vi "Read State.vi"(8 "error in (no error)":errorcluster, 11 "GoalKickKeeperTacticVSS in":refnum<class "GoalKickKeeperTacticVSS.lvclass">) -> (0 "error out":errorcluster, 2 "State":enum16{"GoToBallKeeper", "Kick", "Exit"}(ring), 3 "GoalKickKeeperTacticVSS out":refnum<class "GoalKickKeeperTacticVSS.lvclass">)   [LabVIEW 2023, in "GoalKickKeeperTacticVSS.lvclass"]
uses:
  GoalKickKeeperTacticVSS.lvclass
  GoalKickKeeperTacticVSS.lvclass/GoalKickKeeperTacticVSS.ctl
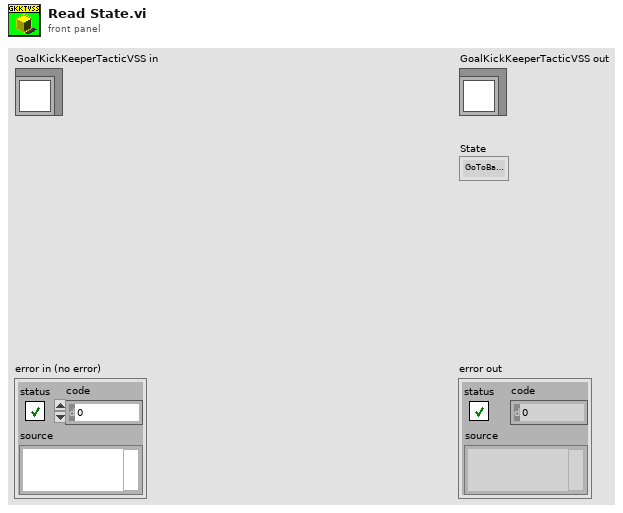
[diagram p1: front panel]
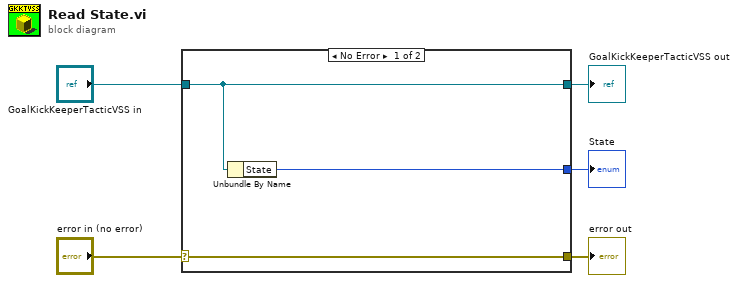
[diagram p0: block diagram]
diagram:
  n1 = case shown="No Error" "error in (no error)" {
    selector: "error in (no error)" -> [w8 w9]
    tunnel: [w8 w9] -> w4
    tunnel: [w7 w10] -> w2
    tunnel: "GoalKickKeeperTacticVSS in" -> [w7 w10]
    tunnel: [w6 _] -> w1
    frame No Error {
      n2 = Unbundle By Name(w7) -> ("State"=w6:enum16{"GoToBallKeeper", "Kick", "Exit"})
    }
    frame Error {
    }
  }
  "error out" <- w4
  "GoalKickKeeperTacticVSS out" <- w2
  "State" <- w1
